vi "HexStringToSingle.vi"(11 "Hex String":string) -> (3 "Single":sgl)   [LabVIEW 2014]
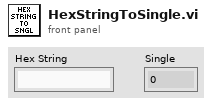
[diagram p1: front panel]
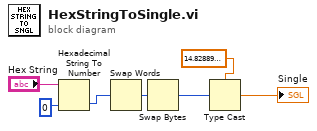
[diagram p0: block diagram]
diagram:
  n1 = Hexadecimal String To Number(string="Hex String", default (0uL)=0 ("default (0 U32)")) -> (number=w3:i32)  [unwired: 1 in, 1 out]
  n2 = Swap Words(1:w3) -> (0:w4:i32)
  n3 = Swap Bytes(anything=w4) -> (byte swapped=w5:i32)
  n4 = Type Cast(type=sgl 14.828897 ("Numeric"), x=w5) -> (*(type *) &x=→"Single":sgl)
